vi "Open.vi"(8 "error in":errorcluster, 9 "isEditable":bool, 10 "Path":path) -> (0 "error out":errorcluster, 3 "SpreadsheetDocument":refnum<k24>)   [LabVIEW 2021, in "Open Xml.lvlib"]
uses:
  Open Xml.lvlib
  D:/git/Open-Xml-LabVIEW/dll/DocumentFormat.OpenXml.dll
  dll/DocumentFormat.OpenXml.dll
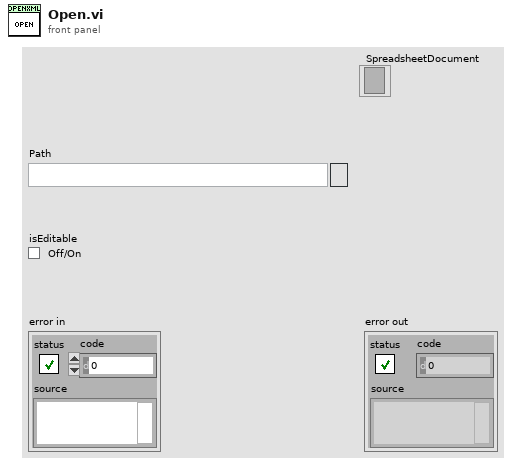
[diagram p1: front panel]
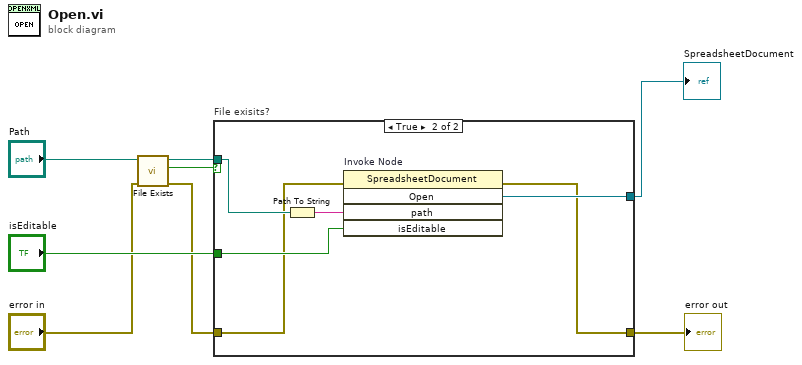
[diagram p0: block diagram]
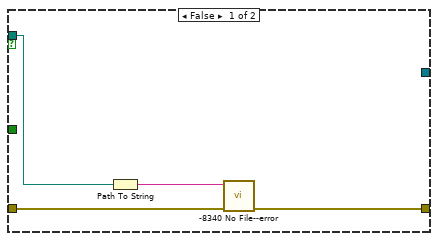
[diagram p2: hidden frame]
diagram:
  n1 = call "File Exists.vi"("error in"="error in", "File Path"="Path") -> ("error out"=w3:errorcluster, "Exists"=w5:bool, "File Path (dup)"=w4:path)  [unwired: 7 in]
  n2 = case "File exisits?" shown="True" w5 {
    tunnel: "isEditable" -> [_ w18]
    tunnel: w4 -> [w10 w17]
    tunnel: w3 -> [w12 w15]
    tunnel: [w11 w13] -> w2
    tunnel: [_ w14] -> w1
    frame False {
      n3 = Path To String(path=w10) -> (string=w9:string)
      n4 = call "-8340 No File--error.vi"("error in (no error)"=w12, "File Path"=w9) -> ("error out"=w11:errorcluster)  [unwired: 9 in]
    }
    frame True {
      n5 = Path To String(path=w17) -> (string=w16:string)
      n6 = invoke on="Invoke Node" class="SpreadsheetDocument" method="Open"(error in=w15, "path"=w16, "isEditable"=w18) -> (error out=w13:errorcluster, "Open"=w14:refnum<k24>)  [unwired: 2 in, 3 out]
    }
  }
  "error out" <- w2
  "SpreadsheetDocument" <- w1
